vi "Waveform.vi"(7 "LabVIEW Web Service Request":refnum<class "Web Request.lvclass">) -> ()   [LabVIEW 2023]
uses:
  <vilib>/wsapi/Web Request.lvclass
panel:
  # "Use the Web Service Request input terminal to call the VIs on the Web Services palette. Do not remove it from the connector pane unless you don't need access to the palette."
  # "Each additional control wired to the connector pane will be available as an input in the URL. To include an indicator in terminal-mode output (the default setting), it must also be wired to the connector pane."
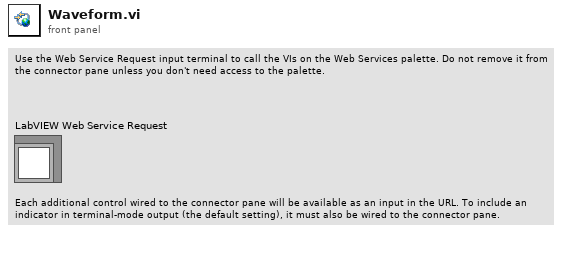
[diagram p1: front panel]
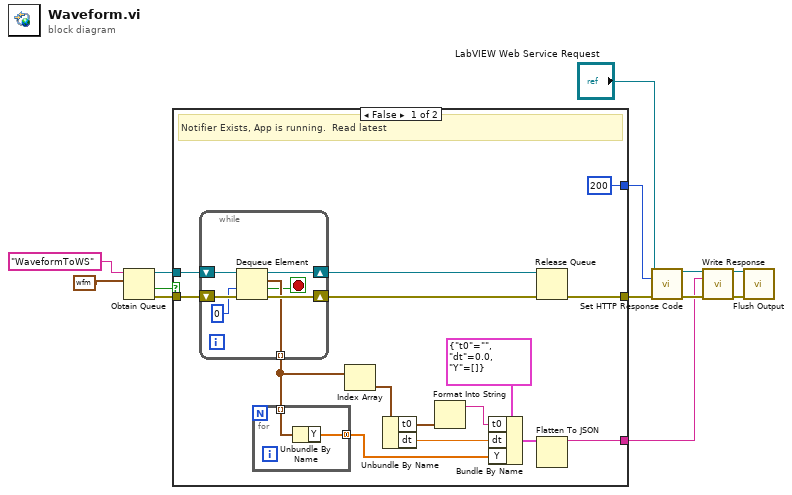
[diagram p0: block diagram]
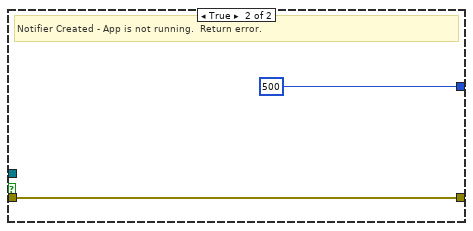
[diagram p2: hidden frame]
diagram:
  n1 = Obtain Queue(name (unnamed)="WaveformToWS", element data type=waveform(dbl) {"t0"=timestamp(0 s since 1904-01-01), "dt"=1.0, "Y"=[]}) -> (queue out=w11:refnum<queue>, created new?=w1:bool, error out=w10:errorcluster)  [unwired: 3 in]
  n2 = case shown="False" w1 {
    tunnel: w11 -> [w27 _]
    tunnel: w10 -> [w26 w39]
    tunnel: [w23 w39] -> w5
    tunnel: [200 500] -> w3
    tunnel: [w19 _] -> w2
    frame False {
      # "Notifier Exists, App is running.  Read latest"
      n3 = while {
        tunnel: [w33] -> w17 mode=indexing
        shift-right: [w34] -> w24
        shift-left: w27 -> [w37]
        shift-right: [w35] -> w25
        shift-left: w26 -> [w36]
        stop <- w31 stop-if-true
        n4 = Dequeue Element(queue=w37, timeout in ms (-1)=0, error in (no error)=w36) -> (queue out=w34:refnum<queue>, element=w33:waveform(dbl), timed out?=w31:bool, error out=w35:errorcluster)
      }
      n5 = for {
        tunnel: w17 -> [w30] mode=indexing
        tunnel: [w29] -> w18 mode=concatenating
        n6 = Unbundle By Name(w30) -> ("Y"=w29:dbl[])
      }
      n7 = Index Array(array=w17) -> (element=w16:waveform(dbl))  [unwired: 1 in]
      n8 = Unbundle By Name(w16) -> ("t0"=w14:timestamp, "dt"=w15:dbl)
      n9 = Format Into String(w14) -> (resulting string=w22:string)  [unwired: 3 in, 1 out]
      n10 = Bundle By Name(cluster=cluster{"t0":string, "dt":dbl, "Y":dbl[]} {"t0"="", "dt"=0.0, "Y"=[]}, "t0"=w22, "dt"=w15, "Y"=w18) -> (w20:cluster{"t0":string, "dt":dbl, "Y":dbl[]})
      n11 = Release Queue(queue=w24, error in (no error)=w25) -> (error out=w23:errorcluster)  [unwired: 1 in, 2 out]
      n12 = Flatten To JSON(anything=w20) -> (JSON string=w19:string)  [unwired: 2 in, 1 out]
    }
    frame True {
      # "Notifier Created - App is not running.  Return error."
    }
  }
  n13 = call <vilib>:"Set HTTP Response Code.vi"("LabVIEW Web Service Request"="LabVIEW Web Service Request", "response code (200)"=w3, "error in (no error)"=w5) -> ("LabVIEW Web Service Request out"=w9:refnum<class "Web Request.lvclass">, "error out"=w8:errorcluster)  [unwired: 11 in]
  n14 = call <vilib>:"Write Response.vi"("LabVIEW Web Service Request"=w9, "response string"=w2, "error in (no error)"=w8) -> ("LabVIEW Web Service Request out"=w7:refnum<class "Web Request.lvclass">, "error out"=w6:errorcluster)  [unwired: 11 in]
  n15 = call <vilib>:"Flush Output.vi"("LabVIEW Web Service Request"=w7, "error in (no error)"=w6) -> ()  [unwired: 12 in, 2 out]
